vi "How to.vi"(8 "Error In":errorcluster) -> (0 "Error Out":errorcluster)   [LabVIEW 2014]
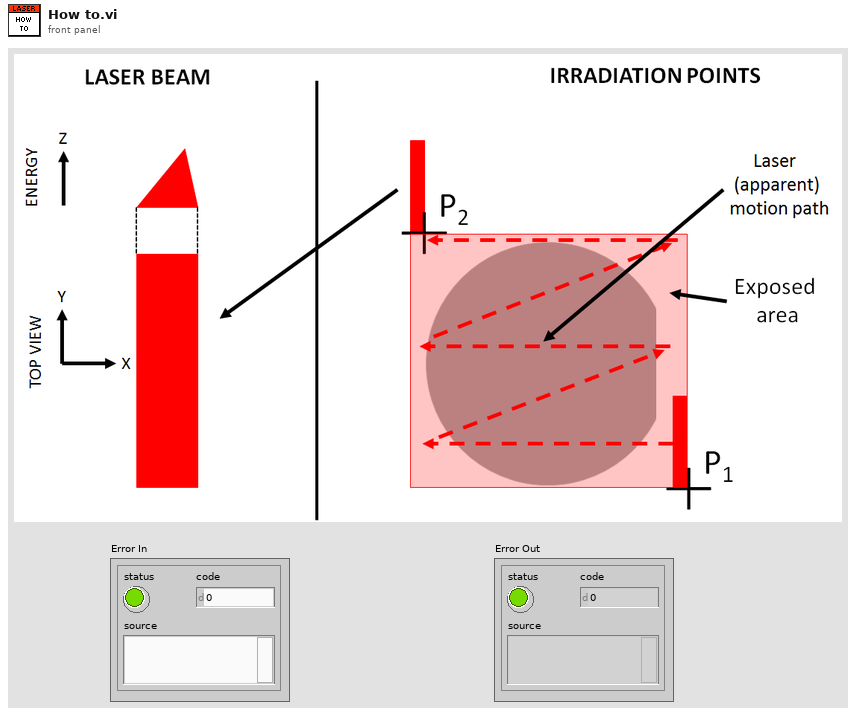
[diagram p1: front panel]
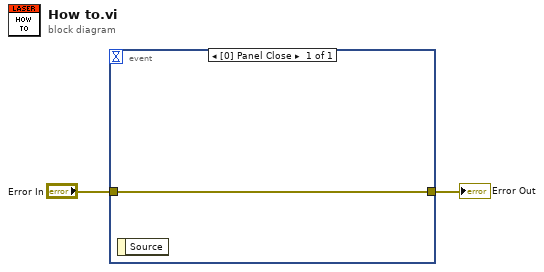
[diagram p0: block diagram]
diagram:
  n1 = event shown="[0] Panel Close" {
    selector: _ -> [_]
    dyn-events: _ -> [_]
    timeout: _ -> [_]
    tunnel: "Error In" -> [w3]
    tunnel: [w3] -> w1
    event Panel Close {
      n2 = event-data() -> ()  [unwired: 1 in, 1 out]
    }
  }
  "Error Out" <- w1
